vi "GeneratePhaseCUDA.vi"() -> ()   [LabVIEW 2019]
uses:
  PCIe16LabVIEWSDK/Interface.dll
panel:
  out "board":i32
  in  "Start SLM":bool
  out "Board ID":i32
  out "# of Boards":i32
  in  "SLM":bool
  in  "Z":dbl(slide) min=-100.0 max=100.0 step=1.0 scale=-100.0..100.0
  out "Delay [ms]":dbl
  out "startCuda Return":i32
  out "Init.":bool
  in  "Y":dbl(slide) min=-100.0 max=100.0 step=1.0 scale=-100.0..100.0
  in  "X":sgl(slide) min=-100 max=100 step=1 scale=-100.0..100.0
  in  "N Iterations":i32=10
  out "N Pixels":i32
  out "SLM Size":i32
  in  "CUDA":bool
  out "stopCUDA Return":i32
  out "generatePhase Return":i32
  out "Path to CUDA DLL":path
  in  "Stop":bool
  out "Phase SLM":T1(plugin-control)
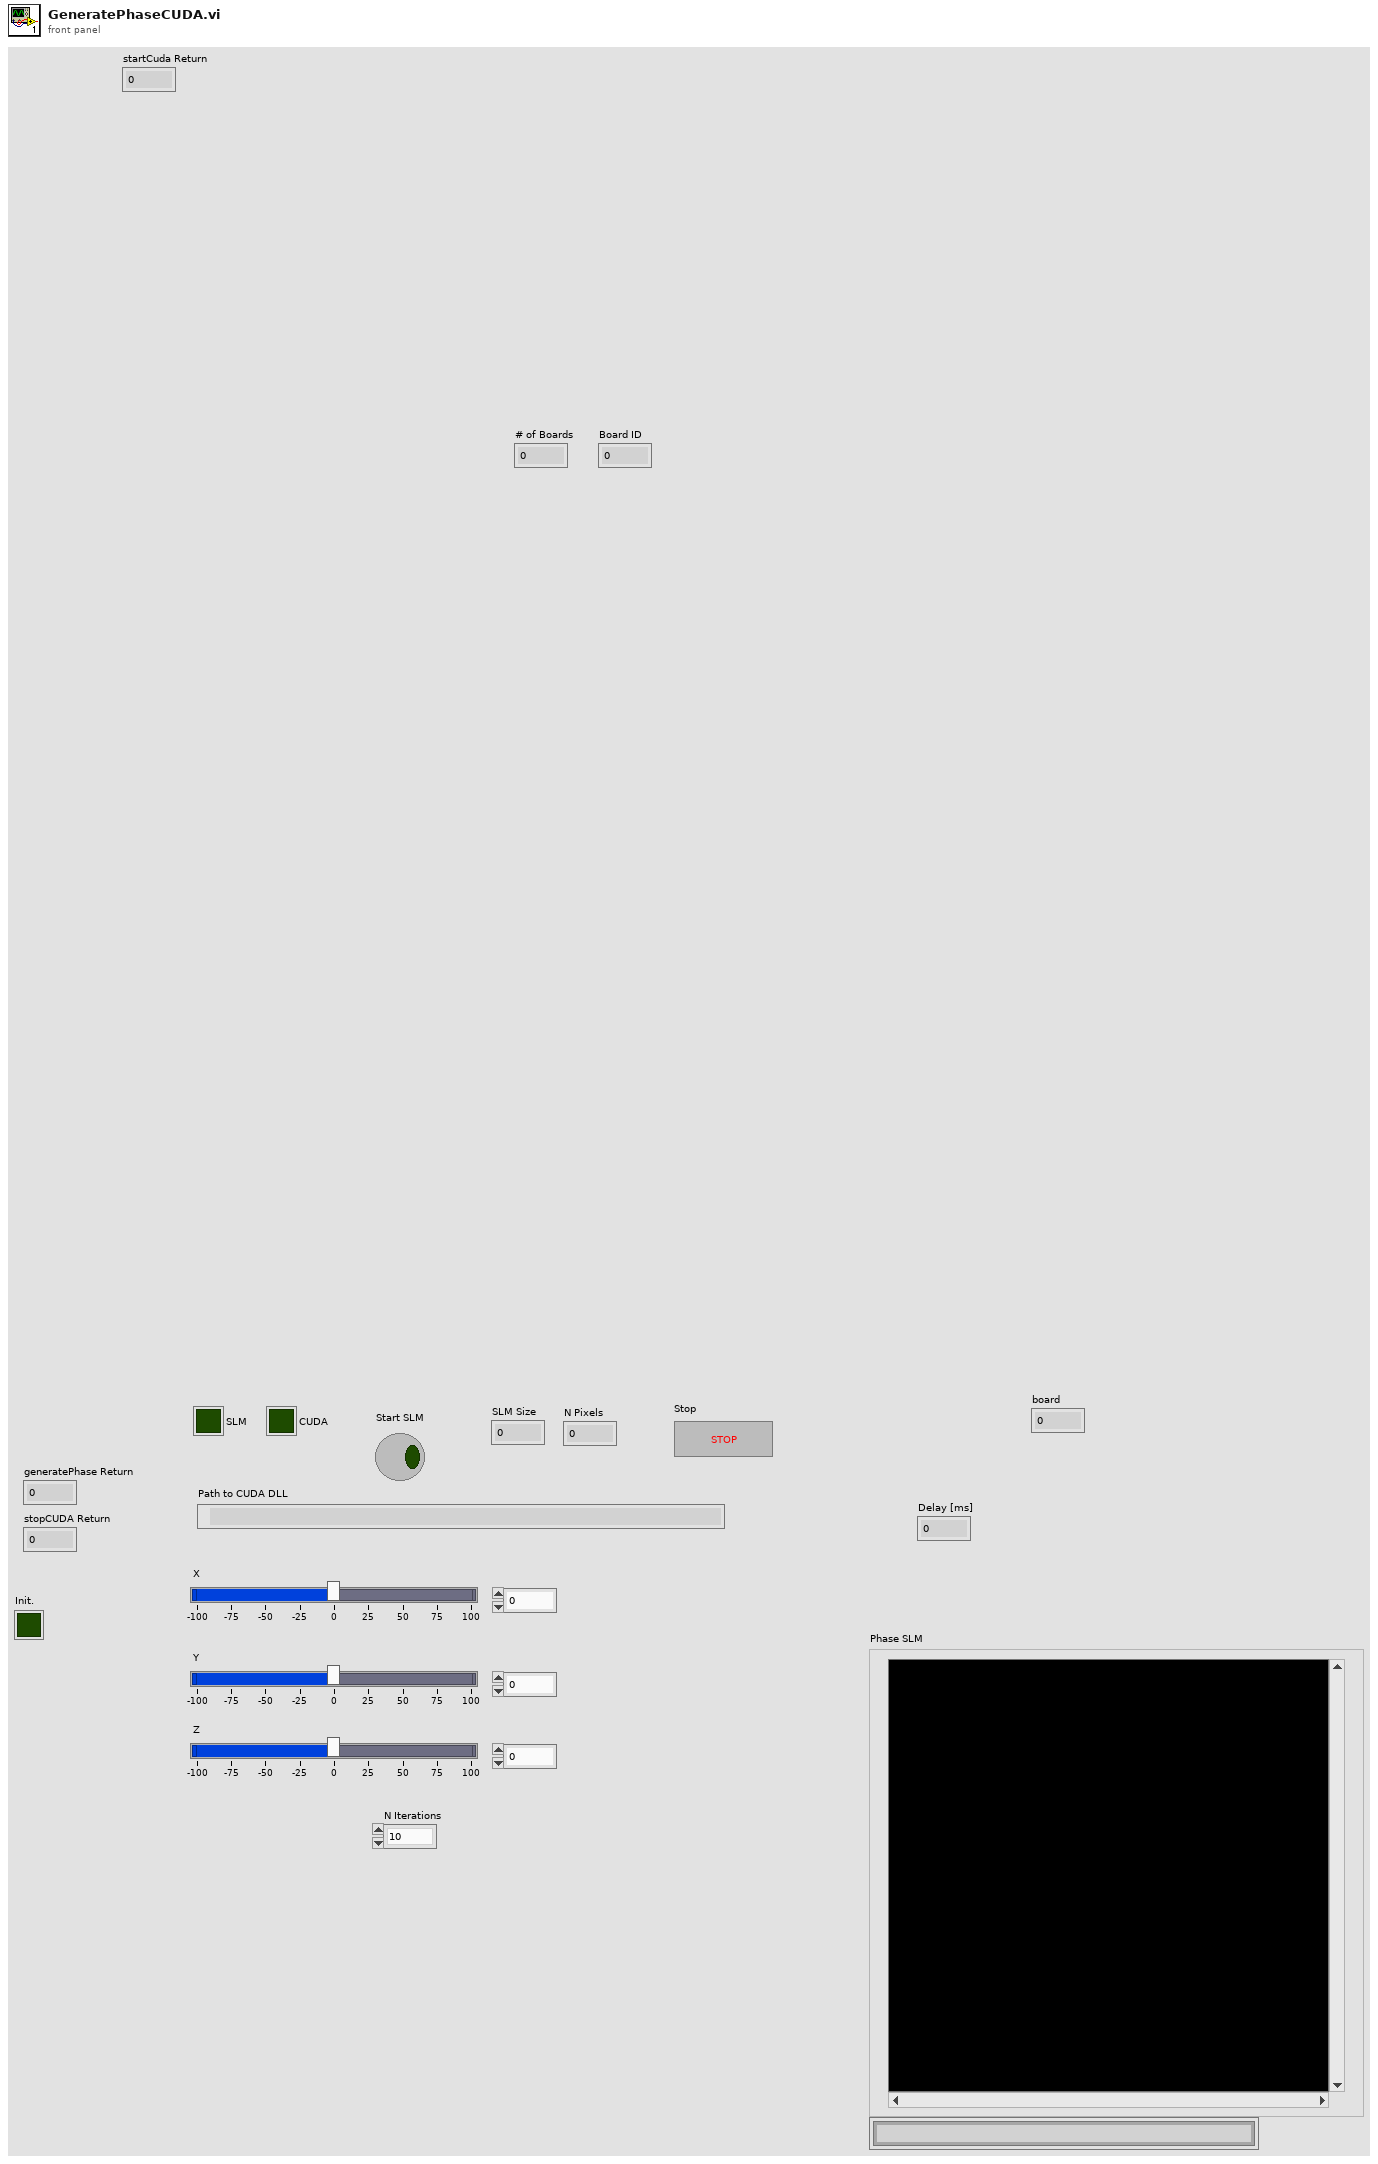
[diagram p1: front panel]
types:
  T1 = typedef "IMAQ Image.ctl" = refnum<image>
  T2 = typedef "Image Type" = u32
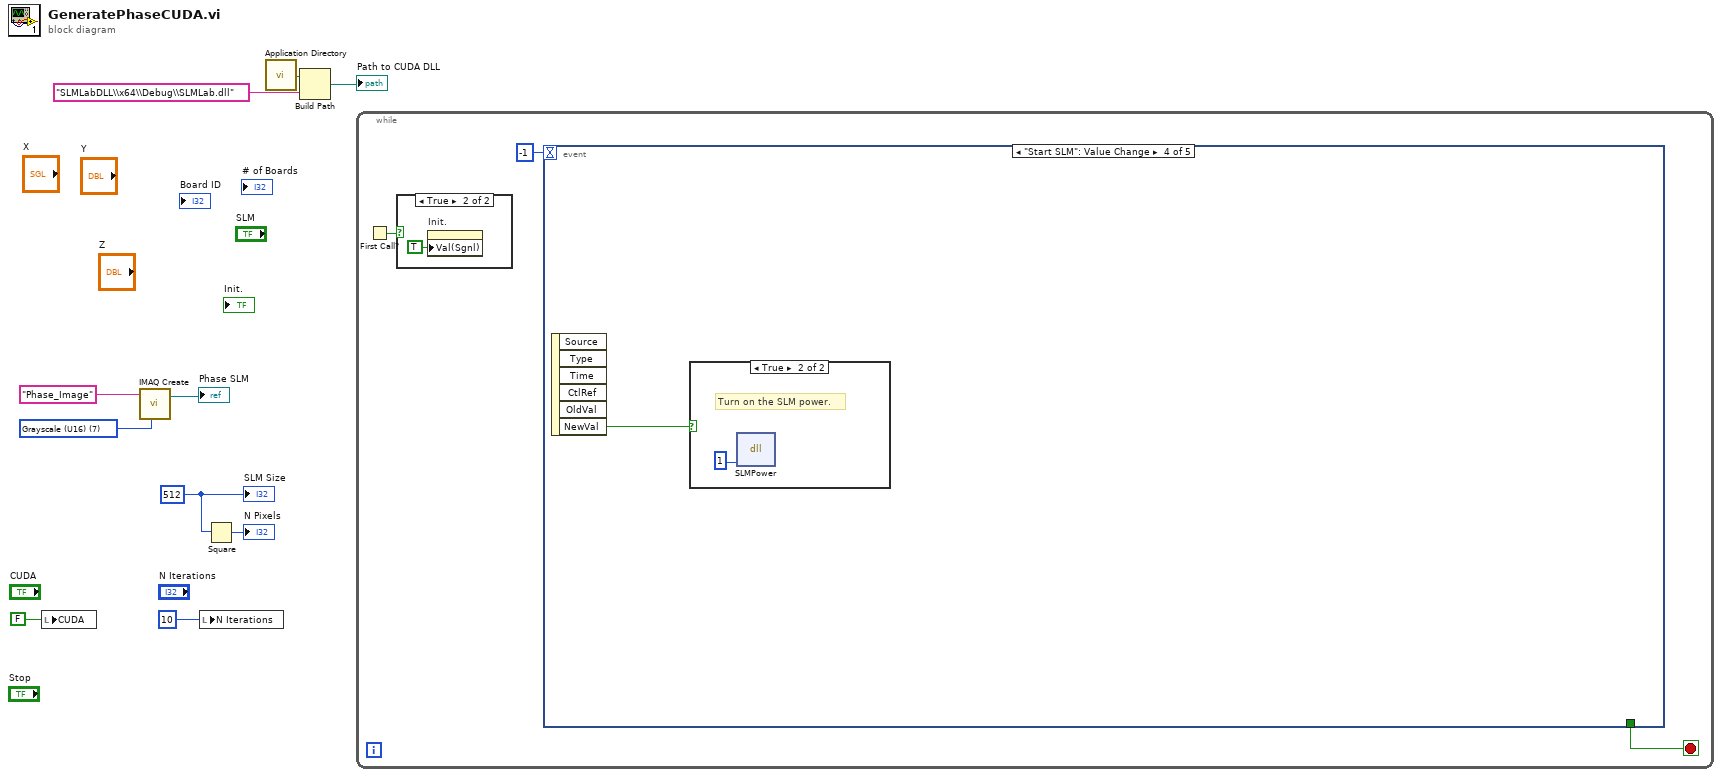
[diagram p0: block diagram]
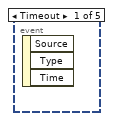
[diagram p3: hidden frame]
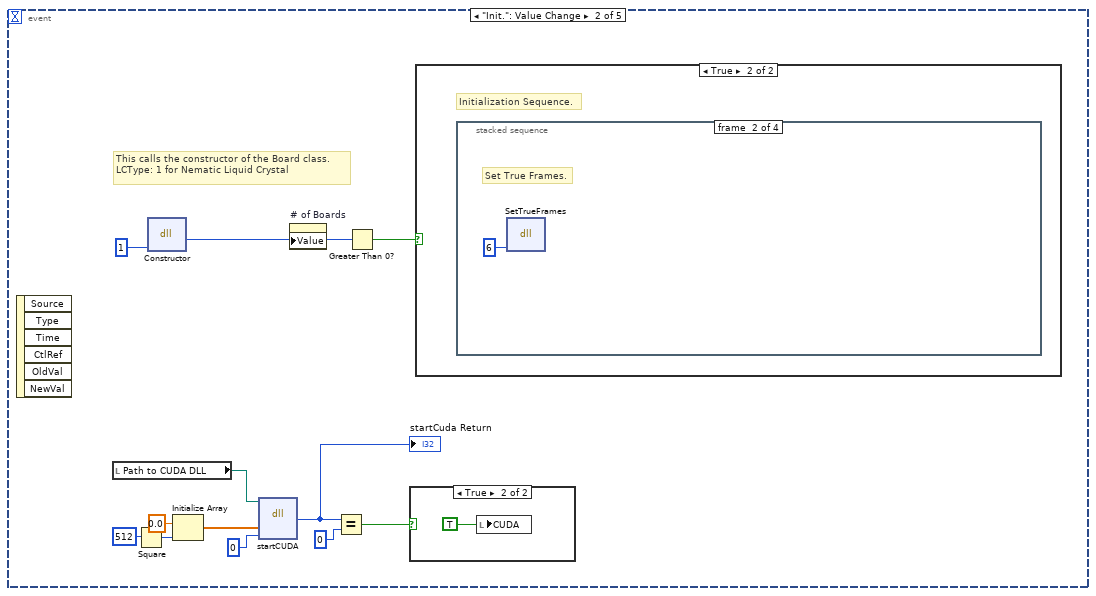
[diagram p4: hidden frame]
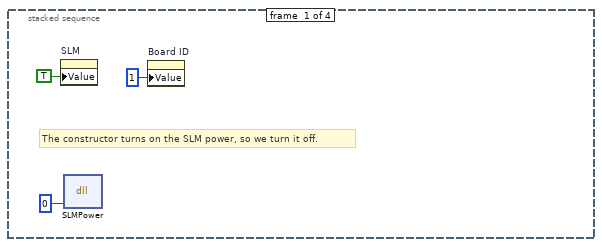
[diagram p6: hidden frame]
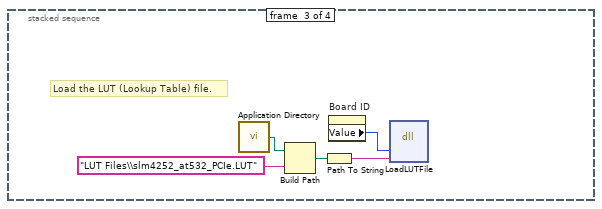
[diagram p7: hidden frame]
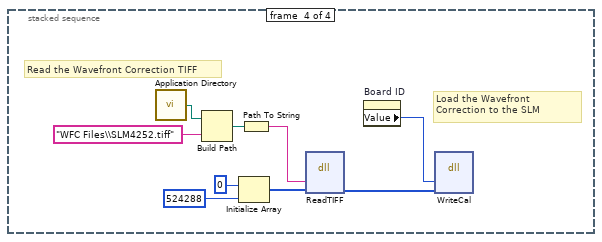
[diagram p8: hidden frame]
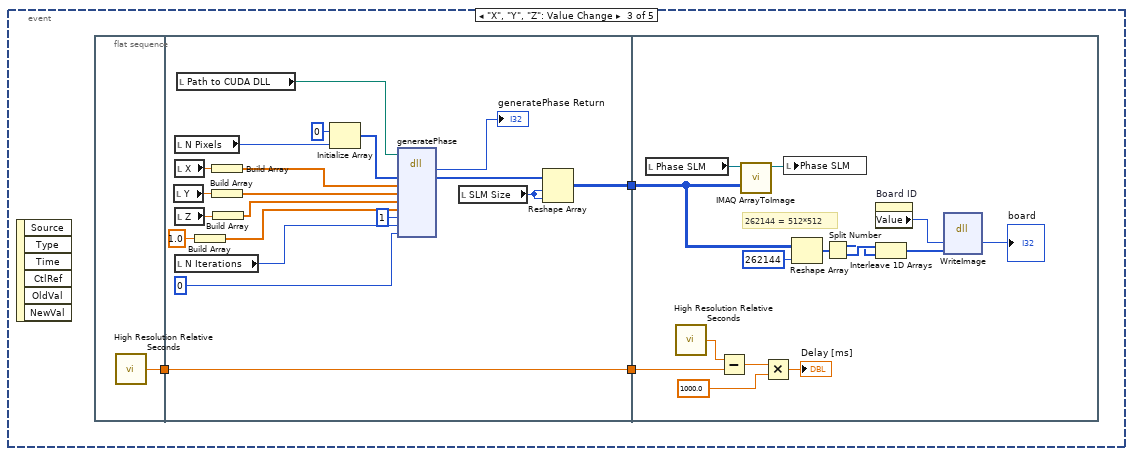
[diagram p10: hidden frame]
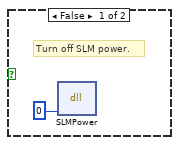
[diagram p11: hidden frame]
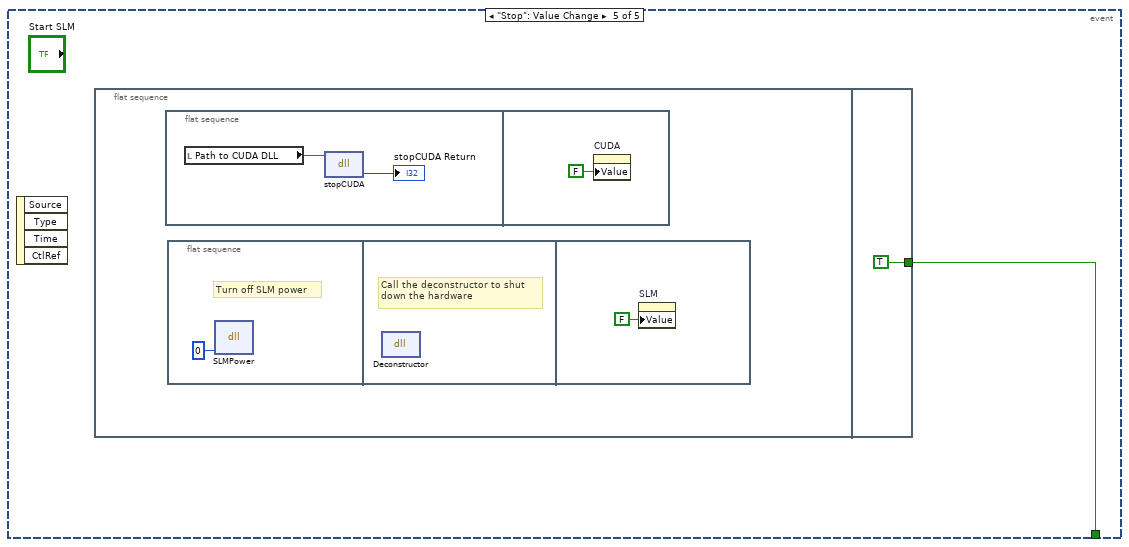
[diagram p12: hidden frame]
diagram:
  w2 = 512
  w9 = T2 7 items=["Grayscale (U8)", "Grayscale (I16)", "Grayscale (SGL)", "Complex (CSG)", "RGB (U32)", "HSL (U32)", "RGB (U64)", "Grayscale (U16)"] ("Image Type")
  n1 = local write "CUDA"(FALSE ("Update SLM")) -> ()
  n2 = call "IMAQ Create"("Image Name"="Phase_Image", "Image Type"=w9) -> ("New Image"=→"Phase SLM":T1)  [unwired: 3 in, 1 out]
  n3 = local write "N Iterations"(10) -> ()
  n4 = Square(x=w2) -> (x^2=→"N Pixels":i32)
  n5 = call <vilib>:"Application Directory.vi"() -> ("Application Directory"=w6:path)
  n6 = Build Path(base path=w6, name or relative path="SLMLabDLL\\x64\\Debug\\SLMLab.dll") -> (appended path=→"Path to CUDA DLL":path)
  n7 = while {
    stop <- w13 stop-if-true
    n8 = First Call?() -> (First Call?: T/F=w11:bool)
    n9 = case shown="True" w11 {
      frame False {
      }
      frame True {
        n10 = property on="Init." class="Bool (strict)"("Val(Sgnl)"=TRUE ("Value (Signaling)")) -> ()  [unwired: 2 in, 2 out]
      }
    }
    n11 = event shown="[3] \"Start SLM\": Value Change" {
      selector: _ -> [_ _ _ _ _]
      dyn-events: _ -> [_ _ _ _ _]
      timeout: -1 -> [_ _ _ _ _]
      tunnel: [_ _ _ _ w88] -> w13
      event Timeout {
        n12 = event-data() -> ()  [unwired: 1 in, 3 out]
      }
      event "Init.": Value Change {
        # "This calls the constructor of the Board class. LCType: 1 for Nematic Liquid Crystal"
        n13 = event-data() -> ()  [unwired: 1 in, 6 out]
        n14 = local read "Path to CUDA DLL"() -> (w24:path)
        n15 = Square(x=512 ("dimension size")) -> (x^2=w22:i32)
        n16 = dll-call lib="C:/PCIe16LabVIEWSDK/Interface.dll" fn="Constructor"("LCType"=u8 1) -> ("return type"=w17:i32)  [unwired: 4 in, 2 out]
        n17 = Initialize Array(sgl 0.0 ("element"), w22) -> (w23:sgl[])
        n18 = dll-call lib="?" fn="startCUDA"(path in=w24, "h_pSLMstart"=w23, "deviceID"=0) -> ("Rückgabetyp"=w25:i32)  [unwired: 4 in, 2 out]
        "startCuda Return" <- w25
        n19 = property on="# of Boards" class="DigNum (strict)"("Value"=w17) -> ()  [unwired: 2 in, 2 out]
        n20 = Equal?(x=w25, y=0) -> (x = y?=w26:bool)
        n21 = Greater Than 0?(x=w17) -> (x > 0?=w16:bool)
        n22 = case shown="True" w26 {
          frame False {
          }
          frame True {
            n23 = local write "CUDA"(TRUE ("Update SLM")) -> ()
          }
        }
        n24 = case shown="True" w16 {
          frame False {
          }
          frame True {
            # "Initialization Sequence."
            n25 = stacked-sequence {
              frame #0 {
                # "The constructor turns on the SLM power, so we turn it off."
                n26 = property on="SLM" class="Bool (strict)"("Value"=TRUE ("SLM")) -> ()  [unwired: 2 in, 2 out]
                n27 = dll-call lib="C:/PCIe16LabVIEWSDK/Interface.dll" fn="SLMPower"("PowerState"=0) -> ()  [unwired: 5 in, 2 out]
                n28 = property on="Board ID" class="DigNum (strict)"("Value"=1 ("Board Number")) -> ()  [unwired: 2 in, 2 out]
              }
              frame #1 {
                # "Set True Frames."
                n29 = dll-call lib="C:/PCIe16LabVIEWSDK/Interface.dll" fn="SetTrueFrames"("TrueFrames"=6) -> ()  [unwired: 5 in, 2 out]
              }
              frame #2 {
                # "Load the LUT (Lookup Table) file."
                n30 = call <vilib>:"Application Directory.vi"() -> ("Application Directory"=w33:path)
                n31 = Build Path(base path=w33, name or relative path="LUT Files\\slm4252_at532_PCIe.LUT") -> (appended path=w34:path)
                n32 = Path To String(path=w34) -> (string=w31:string)
                n33 = property on="Board ID" class="DigNum (strict)"() -> ("Value"=w35:i32)  [unwired: 2 in, 2 out]
                n34 = dll-call lib="C:/PCIe16LabVIEWSDK/Interface.dll" fn="LoadLUTFile"("board"=w35, "LUTPath"=w31) -> ()  [unwired: 6 in, 2 out]
              }
              frame #3 {
                # "Read the Wavefront Correction TIFF"
                # "Load the Wavefront Correction to the SLM"
                n35 = call <vilib>:"Application Directory.vi"() -> ("Application Directory"=w41:path)
                n36 = Build Path(base path=w41, name or relative path="WFC Files\\SLM4252.tiff") -> (appended path=w42:path)
                n37 = Initialize Array(u8 0, 524288) -> (w36:u8[])
                n38 = Path To String(path=w42) -> (string=w39:string)
                n39 = dll-call lib="C:/PCIe16LabVIEWSDK/Interface.dll" fn="ReadTIFF"("TiffPath"=w39, "Image"=w36) -> ("Image"=w44:u8[])  [unwired: 5 in, 2 out]
                n40 = property on="Board ID" class="DigNum (strict)"() -> ("Value"=w43:i32)  [unwired: 2 in, 2 out]
                n41 = dll-call lib="C:/PCIe16LabVIEWSDK/Interface.dll" fn="WriteCal"("board"=w43, "Image"=w44) -> ()  [unwired: 6 in, 2 out]
              }
            }
          }
        }
      }
      event "X", "Y", "Z": Value Change {
        n42 = event-data() -> ()  [unwired: 1 in, 6 out]
        n43 = flat-sequence {
          tunnel: [w49] -> w47
          tunnel: [w52] -> w48
          tunnel: w47 -> [w52]
          tunnel: [w51] -> w46
          tunnel: w48 -> [w84]
          tunnel: w46 -> [w71]
          frame #0 {
            n44 = call <vilib>:"High Resolution Relative Seconds.vi"() -> ("relative seconds"=w49:dbl)
          }
          frame #1 {
            n45 = local read "Y"() -> (w66:dbl)
            n46 = local read "N Pixels"() -> (w61:i32)
            n47 = local read "X"() -> (w64:sgl)
            n48 = local read "Z"() -> (w50:dbl)
            n49 = local read "N Iterations"() -> (w63:i32)
            n50 = local read "Path to CUDA DLL"() -> (w60:path)
            n51 = Build Array(1.0 ("element")) -> (w69:dbl[])
            n52 = Build Array(w64) -> (w65:sgl[])
            n53 = Build Array(w66) -> (w67:dbl[])
            n54 = Build Array(w50) -> (w68:dbl[])
            n55 = Initialize Array(u16 0 ("element"), w61) -> (w59:u16[])
            n56 = dll-call lib="?" fn="generatePhase"(path in=w60, "h_pSLM_uint16"=w59, "x_spots"=w65, "y_spots"=w67, "z_spots"=w68, "I_spots"=w69, "N_spots"=1, "N_interations"=w63, "method"=0) -> ("Return Value"=→"generatePhase Return":i32, "h_pSLM_uint16"=w58:u8[])  [unwired: 9 in, 2 out]
            n57 = local read "SLM Size"() -> (w62:i32)
            n58 = Reshape Array(w58, w62, w62) -> (w51:u8[][])
          }
          frame #2 {
            # "262144 = 512*512"
            n59 = local read "Phase SLM"() -> (w78:T1)
            n60 = call <vilib>:"High Resolution Relative Seconds.vi"() -> ("relative seconds"=w83:dbl)
            n61 = Subtract(x=w83, y=w84) -> (x-y=w82:dbl)
            n62 = call "IMAQ ArrayToImage"("Image Pixels (U16)"=w71, "Image"=w78) -> ("Image Out"=w79:T1)  [unwired: 8 in, 1 out]
            n63 = Multiply(x=w82, y=1000.0) -> (x*y=→"Delay [ms]":dbl)
            n64 = local write "Phase SLM"(w79) -> ()
            n65 = Reshape Array(w71, 262144 ("dimension size")) -> (w76:u8[])
            n66 = Split Number(x=w76) -> (hi(x)=w73:u8[], lo(x)=w74:u8[])
            n67 = property on="Board ID" class="DigNum (strict)"() -> ("Value"=w77:i32)  [unwired: 2 in, 2 out]
            n68 = Interleave 1D Arrays(w74, w73) -> (w75:u8[])
            n69 = dll-call lib="C:/PCIe16LabVIEWSDK/Interface.dll" fn="WriteImage"("board"=w77, "Image"=w75) -> ("board"=→"board":i32)  [unwired: 5 in, 2 out]
          }
        }
      }
      event "Start SLM": Value Change {
        n70 = event-data() -> ("NewVal"=w85:bool)  [unwired: 1 in, 5 out]
        n71 = case shown="True" w85 {
          frame False {
            # "Turn off SLM power."
            n72 = dll-call lib="C:/PCIe16LabVIEWSDK/Interface.dll" fn="SLMPower"("PowerState"=0) -> ()  [unwired: 5 in, 2 out]
          }
          frame True {
            # "Turn on the SLM power."
            n73 = dll-call lib="C:/PCIe16LabVIEWSDK/Interface.dll" fn="SLMPower"("PowerState"=1) -> ()  [unwired: 5 in, 2 out]
          }
        }
      }
      event "Stop": Value Change {
        n74 = event-data() -> ()  [unwired: 1 in, 4 out]
        n75 = flat-sequence {
          tunnel: [TRUE] -> w88
          frame #0 {
            n76 = flat-sequence {
              frame #0 {
                n77 = local read "Path to CUDA DLL"() -> (w89:path)
                n78 = dll-call lib="?" fn="stopCUDA"(path in=w89) -> ("Return Value"=→"stopCUDA Return":i32)  [unwired: 2 in, 2 out]
              }
              frame #1 {
                n79 = property on="CUDA" class="Bool (strict)"("Value"=FALSE ("SLM")) -> ()  [unwired: 2 in, 2 out]
              }
            }
            n80 = flat-sequence {
              frame #0 {
                # "Turn off SLM power"
                n81 = dll-call lib="C:/PCIe16LabVIEWSDK/Interface.dll" fn="SLMPower"("PowerState"=0) -> ()  [unwired: 5 in, 2 out]
              }
              frame #1 {
                # "Call the deconstructor to shut \ndown the hardware"
                n82 = dll-call lib="C:/PCIe16LabVIEWSDK/Interface.dll" fn="Deconstructor"() -> ()  [unwired: 4 in, 2 out]
              }
              frame #2 {
                n83 = property on="SLM" class="Bool (strict)"("Value"=FALSE ("SLM")) -> ()  [unwired: 2 in, 2 out]
              }
            }
          }
          frame #1 {
          }
        }
      }
    }
  }
  "SLM Size" <- w2
